vi "Post-Build Action.vi"(5 "Files Generated by Build":path[](array[path]), 6 "Top Level/Always Included VIs":path[](array[path]), 7 "Destination Path":path, 8 "error in (no error)":errorcluster, 9 "Target Name":string, 10 "Build Specification Name":string, 11 "Project Path":path) -> (0 "error out":errorcluster)   [LabVIEW 2025, in "Example Plugin UI.lvlib"]
uses:
  Example Plugin UI.lvlib
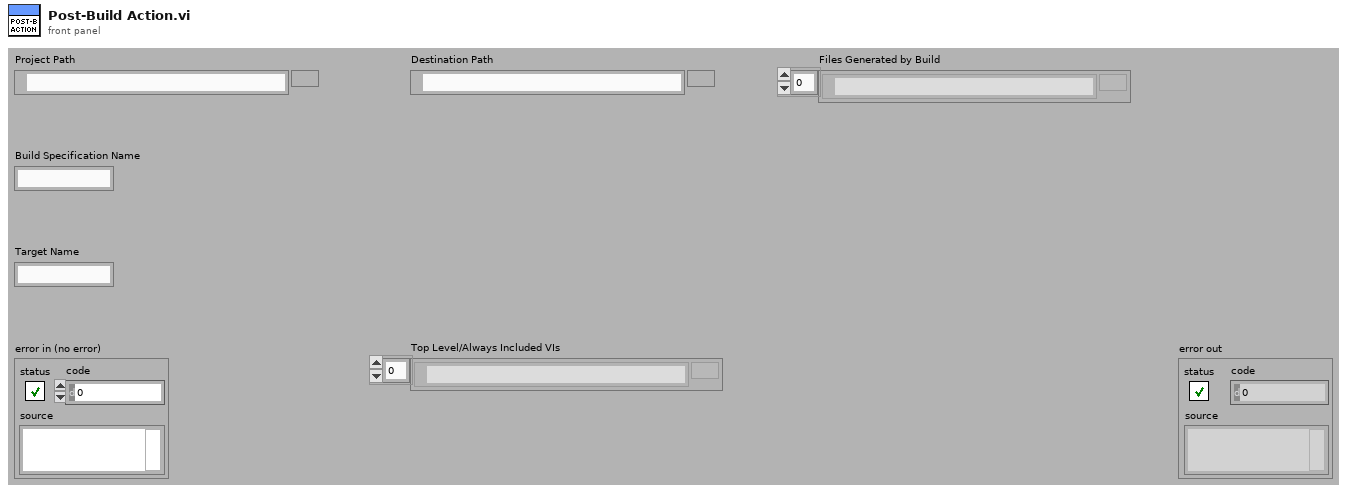
[diagram p1: front panel]
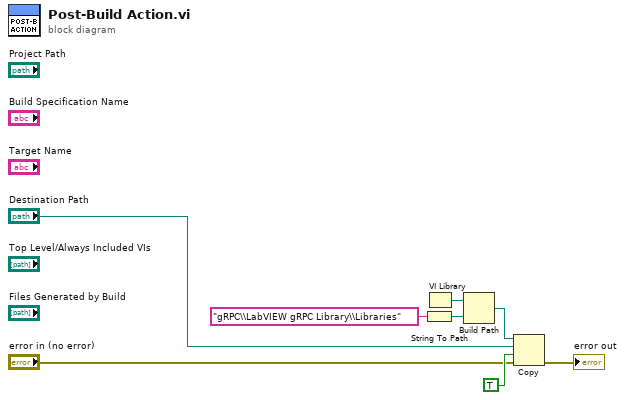
[diagram p0: block diagram]
diagram:
  n1 = String To Path(string="gRPC\\LabVIEW gRPC Library\\Libraries") -> (path=w7:path)
  n2 = VI Library() -> (path=w8:path)
  n3 = Build Path(base path=w8, name or relative path=w7) -> (appended path=w6:path)
  n4 = Copy(8:"error in (no error)", 9:TRUE ("overwrite (F)"), 10:"Destination Path", 11:w6) -> (0:→"error out":errorcluster)  [unwired: 1 in, 2 out]
